vi "compress_messages.vi"(9 "mesage":T1={"time stamp"=timestamp(0 s since 1904-01-01), "object"="", "header"="XX00.XX00.XX00.XX00.XX00", "message"="Z1:00000001000000000200000000030000000004000000000500000000060000000007000000000800000000092345"}, 11 "table":string) -> (3 "message":string)   [LabVIEW 2019, in "PostgreSQL.lvlib"]
uses:
  PostgreSQL.lvlib
  Messages/ctl/LocalMsg.ctl
  Timer Delay/Timers.lvlib
  Messages/Messages.lvlib
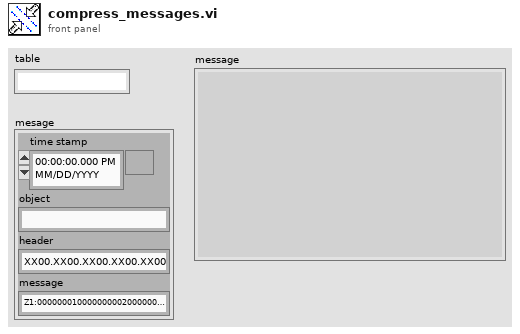
[diagram p1: front panel]
types:
  T1 = typedef "Messages.lvlib/LocalMsg.ctl" = cluster{"time stamp":timestamp, "object":string, "header":string, "message":string}
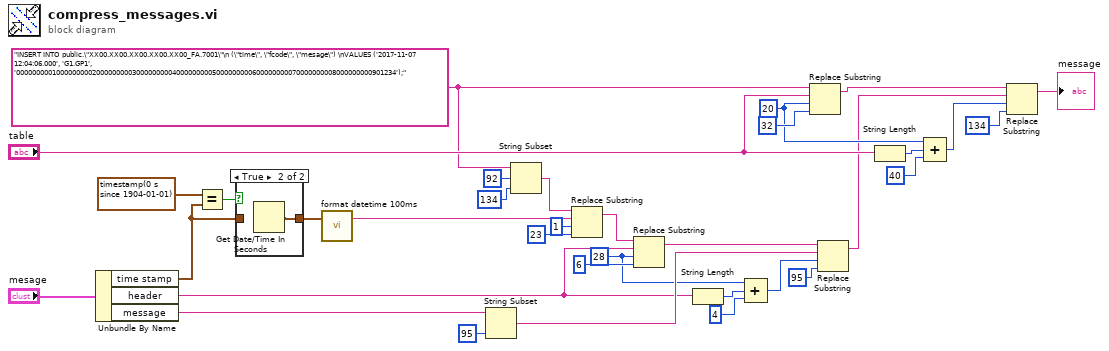
[diagram p0: block diagram]
diagram:
  w10 = 28 ("offset (0)")
  w23 = 20 ("offset (0)")
  w15 = "INSERT INTO public.\"XX00.XX00.XX00.XX00.XX00_FA.7001\"\n (\"time\", \"fcode\", \"mesage\") \nVALUES ('2017-11-07 12:04:06.000', 'G1.GP1', '00000000010000000002000000000300000000040000000005000000000600000000070000000008000000000901234');" ("object 3")
  n1 = Unbundle By Name("mesage") -> ("time stamp"=w3:timestamp, "header"=w11:string, "message"=w14:string)
  n2 = Equal?(x=timestamp(0 s since 1904-01-01), y=w3) -> (x = y?=w2:bool)
  n3 = case shown="True" w2 {
    tunnel: w3 -> [w35 _]
    tunnel: [w35 w36] -> w1
    frame False {
    }
    frame True {
      n4 = Get Date/Time In Seconds() -> (seconds since 1Jan1904=w36:timestamp)
    }
  }
  n5 = call "format datetime 100ms.vi"("time stamp"=w1) -> ("datetime string"=w4:string)  [unwired: 2 in]
  n6 = String Subset(string=w14, length (rest)=95 ("length (rest)")) -> (substring=w18:string)  [unwired: 1 in]
  n7 = String Subset(string=w15, offset (0)=92, length (rest)=134 ("length (rest)")) -> (substring=w24:string)
  n8 = Replace Substring(2:23 ("length (len. of substring)"), 3:1 ("offset (0)"), 4:w4, 5:w24) -> (1:w7:string)  [unwired: 1 out]
  n9 = Replace Substring(2:6 ("x+y"), 3:w10, 4:w11, 5:w7) -> (1:w13:string)  [unwired: 1 out]
  n10 = String Length(string=w11) -> (length=w12:i32)
  n11 = Compound Arithmetic op=ADD(w10, w12, 4 ("value")) -> (w9:i32)
  n12 = Replace Substring(2:32 ("length (len. of substring)"), 3:w23, 4:"table", 5:w15) -> (1:w22:string)  [unwired: 1 out]
  n13 = Replace Substring(2:95 ("x+y"), 3:w9, 4:w18, 5:w13) -> (1:w19:string)  [unwired: 1 out]
  n14 = String Length(string="table") -> (length=w30:i32)
  n15 = Compound Arithmetic op=ADD(w23, w30, 40 ("value")) -> (w28:i32)
  n16 = Replace Substring(2:134 ("length (len. of substring)"), 3:w28, 4:w19, 5:w22) -> (1:→"message":string)  [unwired: 1 out]
